vi "Comunication.vi"() -> ()   [LabVIEW 2018]
doc: "The UDP protocol differs from TCP in that there is no error-checking with the packets of information that are sent, and thus no guarantee whatsoever that an intended recipient will actually receive a given piece of data.\n\nUDP does offer the ability to \"broadcast\" data across a network--simply specify an IP Address of all ones (255.255.255.255) to attempt to broadcast information network-wide. Keep in mind that routers and other network hardware will generally refuse to forward the broadcast beyond certain points, so the extent of the broadcast will in practice be limited."
panel:
  in  "Stop 2":bool
  out "Received Data":dbl(graph)
  in  "Botao 1":bool
  in  "Botao 2":bool
  in  "Stop":bool
  # "Overview: Demonstrates the use of the UDP functions to send data over a UDP connection.\nInstructions:\n1. Run the VI.\n2. Open Simple UDP - Receiver.vi and follow the instructions on its front panel.\n3. Click Stop to stop the VI."
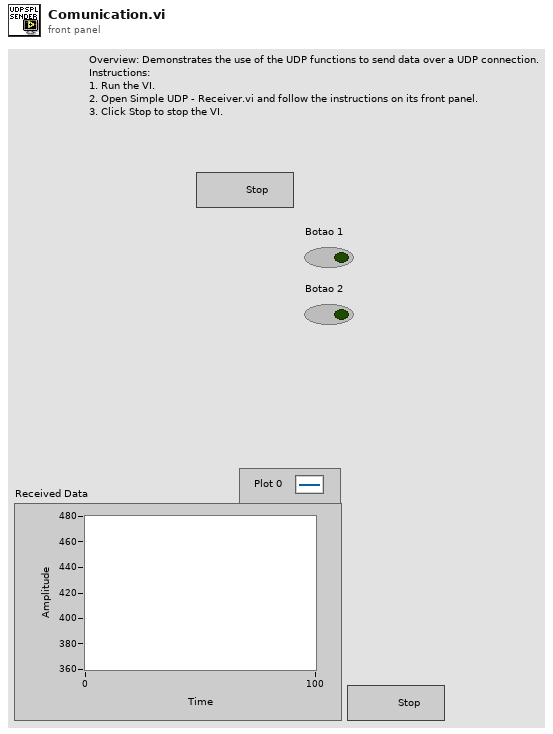
[diagram p1: front panel]
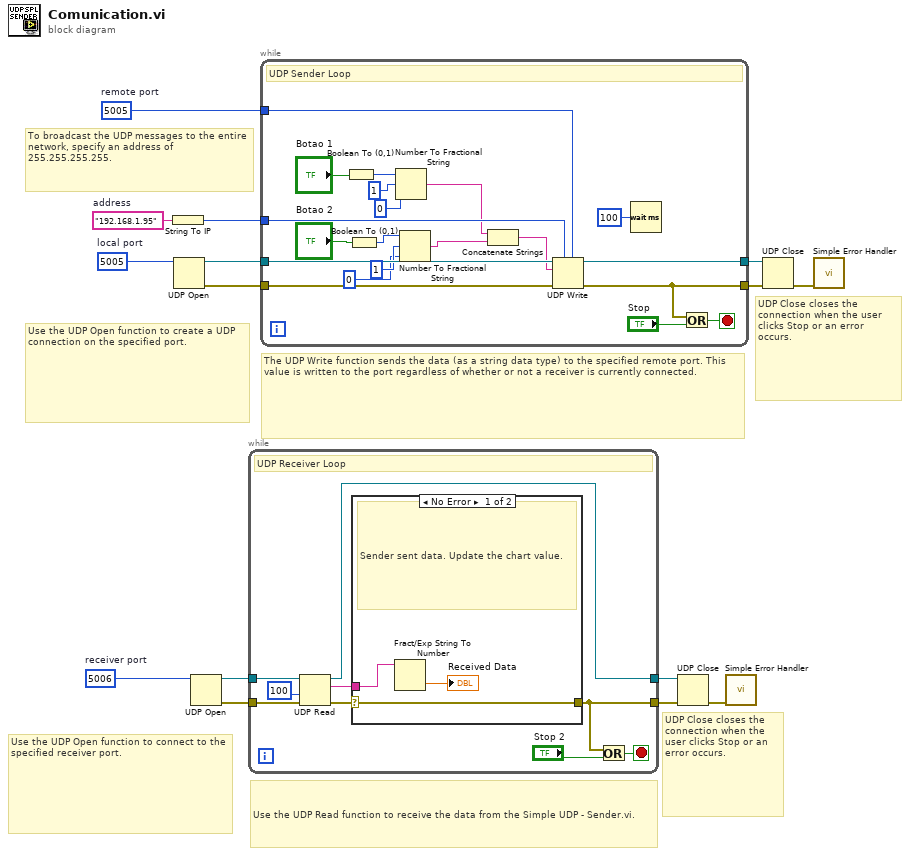
[diagram p0: block diagram]
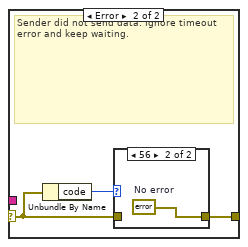
[diagram p2: hidden frame]
diagram:
  w1 = u16 5006  # receiver port
  w7 = u16 5005  # remote port
  w8 = u16 5005  # local port
  w13 = "192.168.1.95"  # address
  # "UDP Close closes the connection when the user clicks Stop or an error occurs."
  # "Use the UDP Open function to connect to the specified receiver port."
  # "Use the UDP Read function to receive the data from the Simple UDP - Sender.vi."
  # "To broadcast the UDP messages to the entire network, specify an address of 255.255.255.255."
  # "UDP Close closes the connection when the user clicks Stop or an error occurs."
  # "The UDP Write function sends the data (as a string data type) to the specified remote port. This value is written to the port regardless of whether or not a receiver is currently connected."
  # "Use the UDP Open function to create a UDP connection on the specified port."
  n1 = String To IP(1:w13) -> (0:w11:u32)
  n2 = UDP Open(11:w8) -> (port=w10:refnum<k16>, 0:w9:errorcluster)  [unwired: 4 in, 1 out]
  n3 = UDP Open(11:w1) -> (port=w2:refnum<k16>, 0:w3:errorcluster)  [unwired: 4 in, 1 out]
  n4 = while {
    tunnel: w2 -> [w24]
    tunnel: [w16] -> w6
    tunnel: w3 -> [w21]
    tunnel: [w17] -> w4
    stop <- w22 stop-if-true
    # "UDP Receiver Loop"
    n5 = UDP Read(connection ID=w24, timeout ms (25000)=100, 8:w21) -> (data out=w19:string, error out=w18:errorcluster, 3:w16:refnum<k16>)  [unwired: 3 out]
    n6 = case shown="No Error" w18 {
      selector: w18 -> [w25 w29]
      tunnel: w19 -> [w27 _]
      tunnel: [w25 w28] -> w17
      frame No Error {
        # "Sender sent data. Update the chart value."
        n7 = Fract/Exp String To Number(string=w27) -> (number=→"Received Data":dbl)  [unwired: 3 in, 1 out]
      }
      frame Error {
        # "Sender did not send data. Ignore timeout error and keep waiting."
        n8 = Unbundle By Name(w29) -> ("code"=w30:i32)
        n9 = case shown="56" w30 {
          tunnel: w29 -> [w31 _]
          tunnel: [w31 w32] -> w28
          frame Default {
          }
          frame 56 {
            w32 = errorcluster {"status"=FALSE, "code"=0, "source"=""}  # No error
          }
        }
      }
    }
    n10 = Or(x=w17, y="Stop 2") -> (x .or. y?=w22:bool)
  }
  n11 = while {
    tunnel: [w47] -> w14
    tunnel: w10 -> [w52]
    tunnel: w9 -> [w51]
    tunnel: [w48] -> w15
    tunnel: w11 -> [w46]
    tunnel: w7 -> [w44]
    stop <- w50 stop-if-true
    # "UDP Sender Loop"
    n12 = Boolean To (0,1)(Boolean="Botao 1") -> (0, 1=w41:i16)
    n13 = Boolean To (0,1)(Boolean="Botao 2") -> (0, 1=w40:i16)
    n14 = Number To Fractional String(number=w41, width (-)=1, precision (6)=0) -> (F-format string=w38:string)  [unwired: 1 in]
    n15 = Number To Fractional String(number=w40, width (-)=1, precision (6)=0) -> (F-format string=w39:string)  [unwired: 1 in]
    n16 = Concatenate Strings(w38, w39) -> (w37:string)
    n17 = UDP Write(address=w46, port or service name=w44, connection ID=w52, data in=w37, 8:w51) -> (error out=w47:errorcluster, 3:w48:refnum<k16>)  [unwired: 1 in]
    n18 = Wait (ms)(milliseconds to wait=u32 100) -> ()  [unwired: 1 out]
    n19 = Or(x=w47, y="Stop") -> (x .or. y?=w50:bool)
  }
  n20 = UDP Close(connection ID=w6, 8:w4) -> (error out=w5:errorcluster)  [unwired: 1 out]
  n21 = call <vilib>:"Simple Error Handler.vi"("error in (no error)"=w5) -> ()  [unwired: 1 in, 8 out]
  n22 = UDP Close(connection ID=w15, 8:w14) -> (error out=w12:errorcluster)  [unwired: 1 out]
  n23 = call <vilib>:"Simple Error Handler.vi"("error in (no error)"=w12) -> ()  [unwired: 4 in, 5 out]
